vi "StandardRelease.vi"(1 "Outgoing Handle":i32, 2 "Incoming Handle":i32) -> ()   [LabVIEW 2013]
uses:
  Madlib.dll
panel:
  # "StandardRelease.vi is meant to be paired with StandardInit.vi for \nuse in VI's that function as a stand-alone VI and as a subVI.\n\nIncoming Handle should be the input of StandardInit.vi.\nOutgoing Handle should be the output of StandardInit.vi."
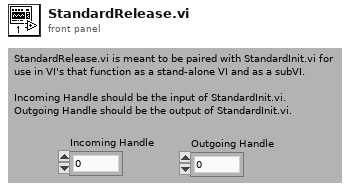
[diagram p1: front panel]
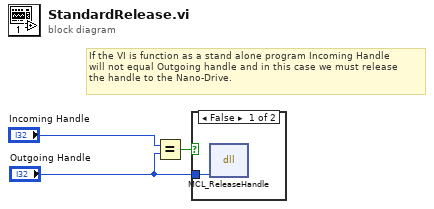
[diagram p0: block diagram]
diagram:
  # "If the VI is function as a stand alone program Incoming Handle \nwill not equal Outgoing handle and in this case we must release\nthe handle to the Nano-Drive."
  n1 = Equal?(x="Incoming Handle", y="Outgoing Handle") -> (x = y?=w3:bool)
  n2 = case shown="False" w3 {
    tunnel: "Outgoing Handle" -> [w4 _]
    frame False {
      n3 = dll-call lib="Z:/Sebastien/LabVIEW/TweezersProjectControl v1/SubVIs_nanostage/MADLib.dll" fn="MCL_ReleaseHandle"("handle"=w4) -> ()  [unwired: 5 in, 2 out]
    }
    frame True {
    }
  }
